vi "API_Get Cursor Position.vi"(8 "错误输入（无错误）":errorcluster) -> (0 "错误输出":errorcluster, 3 "Cursor Pos":cluster{"x":i32, "y":i32})   [LabVIEW 2012, in "API.lvlib"]
doc: "This VI returns the mouse position in screen coordinates."
uses:
  API.lvlib
  user32.dll
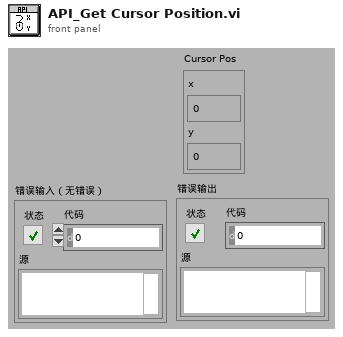
[diagram p1: front panel]
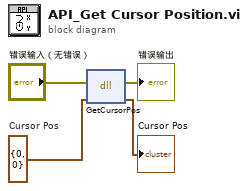
[diagram p0: block diagram]
diagram:
  w4 = cluster{"x":i32, "y":i32} {"x"=0, "y"=0}  # Cursor Pos
  n1 = dll-call lib="user32.dll" fn="GetCursorPos"(error in="错误输入（无错误）", "POINT"=w4) -> (error out=→"错误输出":errorcluster, "POINT"=→"Cursor Pos":cluster{"x":i32, "y":i32})  [unwired: 3 in, 1 out]
